vi "Teleop.vi"(10 "Match Info":T1={"Autonomous Elapsed Seconds"=0.0, "TeleOp Elapsed Seconds"=0.0, "Disabled Elapsed Seconds"=0.0, "Visited Autonomous"=FALSE, "Visited TeleOp"=FALSE, "Visited Disabled"=FALSE, "Autonomous Settings"={"Autonomous Style"=enum."Independent", "VI Refnum"=refnum}}, 11 "Call Context":T2) -> ()   [LabVIEW 2018]
doc: "This VI is called for each TeleOp packet received from the DS where the robot is not disabled. It is often used to read from the joysticks and update I/O or to update setpoints for timed control loops. It should complete and return within 20 milliseconds or it may miss DS packets."
uses:
  <vilib>/Rock Robotics/WPI/DriverStation/WPI_DriverStationDerivedRobotMode.ctl
  <vilib>/Rock Robotics/WPI/DriverStation/WPI_DriverStationMatch Info.ctl
  <vilib>/Rock Robotics/WPI/Solenoid/WPI_SolenoidValue.ctl
  <vilib>/Rock Robotics/WPI/Utilities/WPI_GetSetVariantRefNum.vi
  <vilib>/Rock Robotics/WPI/Solenoid/WPI_SolenoidSetEnum.vi
  <vilib>/Rock Robotics/Network Tables/NT Write Boolean Array.vi
  <vilib>/Rock Robotics/Network Tables/NT Write Numeric Array.vi
  <vilib>/Rock Robotics/Network Tables/NT Read Boolean.vi
  <vilib>/Rock Robotics/Network Tables/NT Read Number.vi
panel:
  out "Sample Slider 0":dbl(slide) scale=0.0..5.0
  out "Sample Boolean 1":bool
  out "Sample Boolean 0":bool
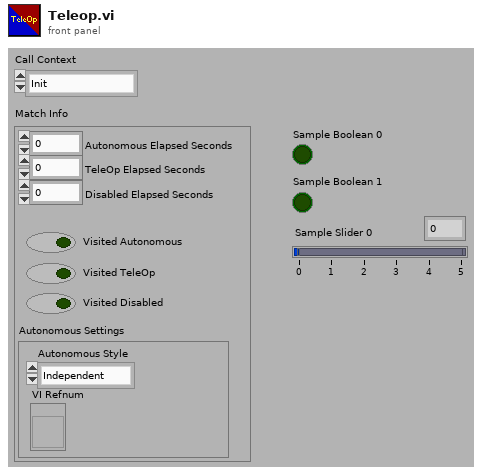
[diagram p1: front panel]
types:
  T1 = typedef "WPI_DriverStationMatch Info.ctl" = cluster{"Autonomous Elapsed Seconds":dbl, "TeleOp Elapsed Seconds":dbl, "Disabled Elapsed Seconds":dbl, "Visited Autonomous":bool, "Visited TeleOp":bool, "Visited Disabled":bool, "Autonomous Settings":cluster{"Autonomous Style":enum16{"Iterative", "Independent"}, "VI Refnum":refnum<vi>}}
  T2 = typedef "WPI_DriverStationDerivedRobotMode.ctl" = enum16{"Init", "Execute", "Stop"}
  T3 = typedef "WPI_RobotDriveDevRef.ctl" = cluster{"DevStatus":errorcluster, "Motors[]":T4[], "Square Inputs":bool, "Max Output":dbl}
  T4 = typedef "WPI_MotorControlDeviceRef.ctl" = cluster{"DeviceStatus":errorcluster, "Type":T5, "PWM":cluster{"PWM Channel":T6, "DeadBand":T7}, "CAN":cluster{"Device Number":u8, "SetOutput VI Ref":variant, "GetOutput VI Ref":variant, "Enable VI Ref":variant, "Disable VI Ref":variant, "Data":variant}, "Invert":bool, "DIO PWM":cluster{"PWM \"Enable\" Channel":T6, "DIOChannel":T8, "PWM Rate":dbl}}
  T5 = typedef "WPI_MotorControlType.ctl" = enum16{"PWM", "CAN", "DIO PWM"}
  T6 = typedef "FPGA_DIOPWMChannel.ctl" = enum8{"PWM 0", "PWM 1", "PWM 2", "PWM 3", "PWM 4", "PWM 5", "PWM 6", "PWM 7", "PWM 8", "PWM 9", "PWM MXP 0", "PWM MXP 1", "PWM MXP 2", "PWM MXP 3", "PWM MXP 4", "PWM MXP 5", "PWM MXP 6", "PWM MXP 7", "PWM MXP 8", "PWM MXP 9", "Invalid"}
  T7 = typedef "WPI_PWMDeadband.ctl" = cluster{"Name":string, "maxPositivePwm":i32, "minPositivePwm":i32, "centerPwm":i32, "maxNegativePwm":i32, "minNegativePwm":i32, "angularRange":u16}
  T8 = typedef "FPGA_DIOChannel.ctl" = enum8{"DIO 0", "DIO 1", "DIO 2", "DIO 3", "DIO 4", "DIO 5", "DIO 6", "DIO 7", "DIO 8", "DIO 9", "DIO MXP 0", "DIO MXP 1", "DIO MXP 2", "DIO MXP 3", "DIO MXP 4", "DIO MXP 5", "DIO MXP 6", "DIO MXP 7", "DIO MXP 8", "DIO MXP 9", "DIO MXP 10", "DIO MXP 11", "DIO MXP 12", "DIO MXP 13", "DIO MXP 14", "DIO MXP 15", "SPI Port CS1", "SPI Port CS2", "SPI Port CS3", "SPI Port MISO", "SPI Port MOSI", "Invalid"}
  T9 = typedef "WPI_JoystickDevRef.ctl" = cluster{"Device":T10}
  T10 = typedef "WPI_JoystickDeviceEnum.ctl" = enum16{"USB 0", "USB 1", "USB 2", "USB 3", "USB 4", "USB 5"}
  T11 = typedef "WPI_SolenoidValue.ctl" = enum16{"Off", "On", "Forward", "Reverse"}
  T12 = typedef "WPI_SolenoidDevRef.ctl" = cluster{"DevStatus":errorcluster, "Pneumatics Control Module":u8, "Forward Solenoid Channel":T13, "Reverse Solenoid Channel":T13}
  T13 = typedef "WPI_SolenoidChannel.ctl" = enum8{"Solenoid 0", "Solenoid 1", "Solenoid 2", "Solenoid 3", "Solenoid 4", "Solenoid 5", "Solenoid 6", "Solenoid 7", "Invalid"}
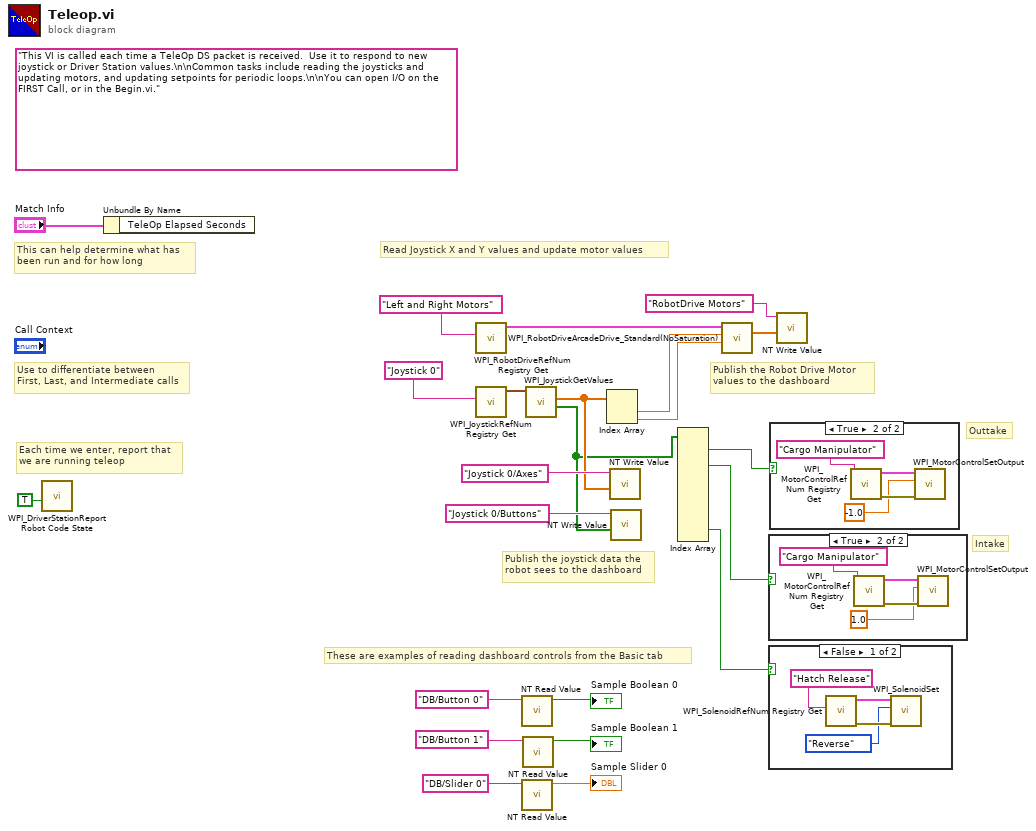
[diagram p0: block diagram]
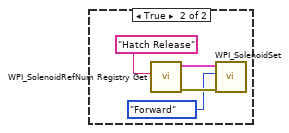
[diagram p2: hidden frame]
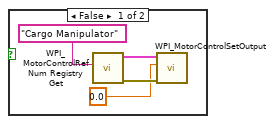
[diagram p3: hidden frame]
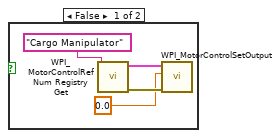
[diagram p4: hidden frame]
diagram:
  (unwired) "This VI is called each time a TeleOp DS packet is received.  Use it to respond to new joystick or Driver Station values.\n\nCommon tasks include reading the joysticks and updating motors, and updating setpoints for periodic loops.\n\nYou can open I/O on the FIRST Call, or in the Begin.vi."
  # "Intake"
  # "Outtake"
  # "These are examples of reading dashboard controls from the Basic tab"
  # "Publish the Robot Drive Motor\nvalues to the dashboard"
  # "Publish the joystick data the\nrobot sees to the dashboard"
  # "Each time we enter, report that\nwe are running teleop"
  # "Use to differentiate between\nFirst, Last, and Intermediate calls"
  # "This can help determine what has\nbeen run and for how long"
  # "Read Joystick X and Y values and update motor values"
  n1 = call <vilib>:"WPI_DriverStationReport Robot Code State.vi"("TeleOp"=TRUE ("Autonomous")) -> ()  [unwired: 10 in, 1 out]
  n2 = Unbundle By Name("Match Info") -> ()  [unwired: 1 out]
  n3 = call <vilib>:"WPI_RobotDriveRefNum Registry Get.vi"("refnum name"="Left and Right Motors") -> ("RobotDriveDevRef"=w21:T3)  [unwired: 1 in, 9 out]
  n4 = call <vilib>:"WPI_JoystickRefNum Registry Get.vi"("refnum name"="Joystick 0") -> ("JoystickDevRef"=w18:T9)  [unwired: 1 in, 9 out]
  n5 = call-poly <vilib>:"NT Read Value.vi"("Name"="DB/Button 0" ("refnum name")) -> ("Boolean"=→"Sample Boolean 0":bool)  [unwired: 9 in, 1 out]
  n6 = call-poly <vilib>:"NT Read Value.vi"("Name"="DB/Slider 0" ("refnum name")) -> ("Numeric"=→"Sample Slider 0":dbl)  [unwired: 9 in, 1 out]
  n7 = call-poly <vilib>:"NT Read Value.vi"("Name"="DB/Button 1" ("refnum name")) -> ("Boolean"=→"Sample Boolean 1":bool)  [unwired: 9 in, 1 out]
  n8 = call <vilib>:"WPI_JoystickGetValues.vi"("JoystickDevRef"=w18) -> ("Buttons"=w4:bool[], "Axes"=w13:dbl[])  [unwired: 6 in, 3 out]
  n9 = Index Array(array=w13) -> (element #1=w20:dbl, element #2=w16:dbl)  [unwired: 2 in]
  n10 = call-poly <vilib>:"NT Write Value.vi"("Numeric Array"=w13, "Name"="Joystick 0/Axes") -> ()  [unwired: 9 in, 1 out]
  n11 = call-poly <vilib>:"NT Write Value.vi"("Boolean Array"=w4, "Name"="Joystick 0/Buttons") -> ()  [unwired: 9 in, 1 out]
  n12 = Index Array(array=w4) -> (element #1=w3:bool, element #3=w2:bool, element #11=w1:bool)  [unwired: 12 in, 9 out]
  n13 = call <vilib>:"WPI_RobotDriveArcadeDrive_Standard(NoSaturation).vi"("Y axis value"=w16, "X axis value"=w20, "RobotDriveDevRef"=w21) -> ("Motor Values"=w6:dbl[])  [unwired: 1 in, 7 out]
  n14 = case shown="True" w2 {
    frame False {
      n15 = call <vilib>:"WPI_MotorControlRefNum Registry Get.vi"("refnum name"="Cargo Manipulator") -> ("error out"=w27:errorcluster, "MotorControlDevRef"=w26:T4)  [unwired: 9 in]
      n16 = call <vilib>:"WPI_MotorControlSetOutput.vi"("error in (no error)"=w27, "Output"=0.0, "MotorControlDevRef"=w26) -> ()  [unwired: 6 in, 3 out]
    }
    frame True {
      n17 = call <vilib>:"WPI_MotorControlRefNum Registry Get.vi"("refnum name"="Cargo Manipulator") -> ("error out"=w30:errorcluster, "MotorControlDevRef"=w31:T4)  [unwired: 9 in]
      n18 = call <vilib>:"WPI_MotorControlSetOutput.vi"("error in (no error)"=w30, "Output"=1.0, "MotorControlDevRef"=w31) -> ()  [unwired: 6 in, 3 out]
    }
  }
  n19 = case shown="False" w1 {
    frame False {
      n20 = call <vilib>:"WPI_SolenoidRefNum Registry Get.vi"("refnum name"="Hatch Release") -> ("error out"=w33:errorcluster, "SolenoidDevRef"=w34:T12)  [unwired: 9 in]
      n21 = call-poly <vilib>:"WPI_SolenoidSet.vi"("error in (no error)"=w33, "Value"=WPI_SolenoidValue."Reverse", "SolenoidDevRef"=w34) -> ()  [unwired: 7 in, 2 out]
    }
    frame True {
      n22 = call <vilib>:"WPI_SolenoidRefNum Registry Get.vi"("refnum name"="Hatch Release") -> ("error out"=w37:errorcluster, "SolenoidDevRef"=w38:T12)  [unwired: 9 in]
      n23 = call-poly <vilib>:"WPI_SolenoidSet.vi"("error in (no error)"=w37, "Value"=WPI_SolenoidValue."Forward", "SolenoidDevRef"=w38) -> ()  [unwired: 7 in, 2 out]
    }
  }
  n24 = case shown="True" w3 {
    frame False {
      n25 = call <vilib>:"WPI_MotorControlRefNum Registry Get.vi"("refnum name"="Cargo Manipulator") -> ("error out"=w42:errorcluster, "MotorControlDevRef"=w43:T4)  [unwired: 9 in]
      n26 = call <vilib>:"WPI_MotorControlSetOutput.vi"("error in (no error)"=w42, "Output"=0.0, "MotorControlDevRef"=w43) -> ()  [unwired: 6 in, 3 out]
    }
    frame True {
      n27 = call <vilib>:"WPI_MotorControlRefNum Registry Get.vi"("refnum name"="Cargo Manipulator") -> ("error out"=w46:errorcluster, "MotorControlDevRef"=w47:T4)  [unwired: 9 in]
      n28 = call <vilib>:"WPI_MotorControlSetOutput.vi"("error in (no error)"=w46, "Output"=-1.0, "MotorControlDevRef"=w47) -> ()  [unwired: 6 in, 3 out]
    }
  }
  n29 = call-poly <vilib>:"NT Write Value.vi"("Numeric Array"=w6, "Name"="RobotDrive Motors") -> ()  [unwired: 9 in, 1 out]
